vi "Get Active Numeric Function.vi"(0 "Numeric Functions in":refnum<class "Array Functions.lvclass">, 11 "error in (no error)":errorcluster) -> (4 "Numeric Functions out":refnum<class "Array Functions.lvclass">, 6 "Function":T1, 15 "error out":errorcluster)   [LabVIEW 2019, in "Array Functions.lvclass"]
uses:
  Array Functions.lvclass
  C:/Users/Patrick/Documents/GitHub/LabVIEW-Script-Language/source code/LSL components/functions/functionsbase/functionbase.lvclass
  Function List.ctl
  functionsbase/functionbase.lvclass
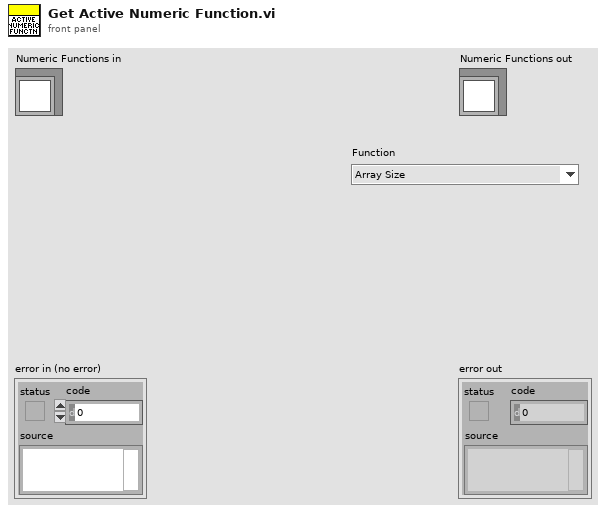
[diagram p1: front panel]
types:
  T1 = typedef "Array Functions.lvclass/Function List.ctl" = enum16{"Array Size", "Index Array", "Replace Subset", "Insert Into Array", "Delete From Array", "Initialize 1D Array", "Initialize 2D Array", "Build Array", "Array Subset", "Max in Array", "Min in Array", "Sort 1D Array", "Search 1D Aray", "Reverse 1D Array", "Slice by start stop", "Slice by start stop step", "range by start stop", "range by start stop step"}
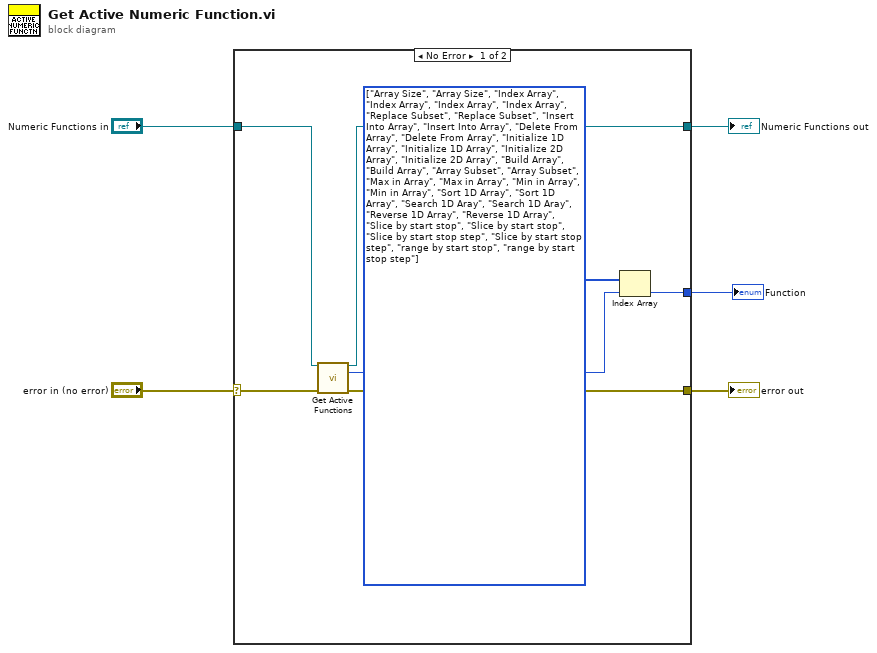
[diagram p0: block diagram]
diagram:
  n1 = case shown="No Error" "error in (no error)" {
    selector: "error in (no error)" -> [w10 w14]
    tunnel: [w8 w14] -> w4
    tunnel: [w7 w13] -> w2
    tunnel: "Numeric Functions in" -> [w9 w13]
    tunnel: [w11 _] -> w1
    frame No Error {
      w12 = T1[] [enum."Array Size", enum."Array Size", enum."Index Array", enum."Index Array", enum."Index Array", enum."Index Array", enum."Replace Subset", enum."Replace Subset", enum."Insert Into Array", enum."Insert Into Array", enum."Delete From Array", enum."Delete From Array", enum."Initialize 1D Array", enum."Initialize 1D Array", enum."Initialize 2D Array", enum."Initialize 2D Array", enum."Build Array", enum."Build Array", enum."Array Subset", enum."Array Subset", enum."Max in Array", enum."Max in Array", enum."Min in Array", enum."Min in Array", enum."Sort 1D Array", enum."Sort 1D Array", enum."Search 1D Aray", enum."Search 1D Aray", enum."Reverse 1D Array", enum."Reverse 1D Array", enum."Slice by start stop", enum."Slice by start stop", enum."Slice by start stop step", enum."Slice by start stop step", enum."range by start stop", enum."range by start stop step"] items=["Array Size", "Index Array", "Replace Subset", "Insert Into Array", "Delete From Array", "Initialize 1D Array", "Initialize 2D Array", "Build Array", "Array Subset", "Max in Array", "Min in Array", "Sort 1D Array", "Search 1D Aray", "Reverse 1D Array", "Slice by start stop", "Slice by start stop step", "range by start stop", "range by start stop step"]
      n2 = call "Get Active Functions.vi"("functionbase in"=w9, "error in (no error)"=w10) -> ("functionbase out"=w7:refnum<class "Array Functions.lvclass">, "Syntax Index"=w6:i32, "error out"=w8:errorcluster)  [unwired: 11 in]
      n3 = Index Array(array=w12, index=w6) -> (element=w11:T1)
    }
    frame Error {
    }
  }
  "error out" <- w4
  "Numeric Functions out" <- w2
  "Function" <- w1
